vi "UCL_Query.vi"(0 "System no.":i32=1 min=1 max=4 step=1, 5 "error in":errorcluster) -> (14 "Command Level":T1, 19 "error out":errorcluster)   [LabVIEW 2020]
doc: "UCL? (Get User Command Level) \n\nDescription\nReads the active user command level for the GCS interpreter of the communication interface \nused.\nThe active user command level of the GCS interpreter determines which commands are \navailable on the interface and for which parameters read and write access is granted.\n\nFormat\nUCL?\n\nArguments\nnone\n\nResponse\n<User Command Level> is the user command level that is currently active in the GCS interpreter \nof the communication interface used.\nPermissions and passwords for the individual user command levels:\nUser command level Permissions Password\nUSR User Level\nAccessible are functionalities for normal operation \nand settings that must be adjustable in normal \noperation (e.g. parameters for adjusting the control \ncharacteristics).\nNo password \nrequired\nADV Expert Customer\nAccessible are the functionalities and settings of the \nlevel USR as well as all parameters and commands \nthe user needs for the configuration\nADVANCED\nFAY Only PI Staff\nPI-internal use\n-\nDEV Only FW Developers\nPI-internal use\n-\n\nUser command level\nUSR"
uses:
  UserCommandLevel.ctl
panel:
  # "UCL? (Get User Command Level) \n\nReads the active user command level for the GCS interpreter of the communication interface \nused.\nThe active user command level of the GCS interpreter determines which commands are \navailable on the interface and for which parameters read and write access is granted."
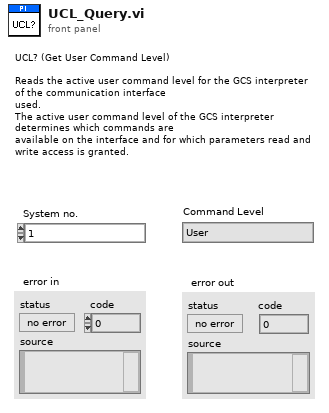
[diagram p1: front panel]
types:
  T1 = typedef "UserCommandLevel.ctl" = enum16{"User", "Expert", "PI Staff", "FW Developer"}
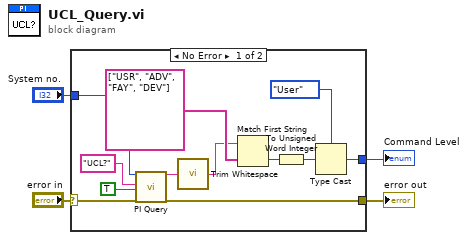
[diagram p0: block diagram]
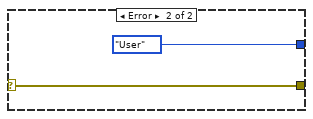
[diagram p2: hidden frame]
diagram:
  n1 = case shown="No Error" "error in" {
    selector: "error in" -> [w16 w18]
    tunnel: [w10 w18] -> w4
    tunnel: "System no." -> [w15 _]
    tunnel: [w12 UserCommandLevel."User" ("Command Level")] -> w1
    frame No Error {
      n2 = call "PI Query.vi"("System no."=w15, "String to send"="UCL?", "Attach termination char.?"=TRUE, "error in"=w16) -> ("String read"=w7:string, "error out"=w10:errorcluster)  [unwired: 12 in, 2 out]
      n3 = call "Trim Whitespace.vi"("string"=w7) -> ("trimmed string"=w8:string)  [unwired: 1 in]
      n4 = Match First String(2:string[] ["USR", "ADV", "FAY", "DEV"], 3:w8) -> (0:w6:i32)  [unwired: 1 out]
      n5 = To Unsigned Word Integer(number=w6) -> (unsigned 16bit integer=w5:u16)
      n6 = Type Cast(type=UserCommandLevel."User" ("Command Level"), x=w5) -> (*(type *) &x=w12:T1)
    }
    frame Error {
    }
  }
  "error out" <- w4
  "Command Level" <- w1
